vi "TP 2.3 (con variable t).vi"() -> ()   [LabVIEW 2013]
panel:
  in  "Función":T1(ring)
  in  "stop":bool
  out "Waveform Graph":dbl[](graph)
  in  "Amplitud":dbl
  in  "Frecuencia":dbl
  in  "Cantida de Muestras":dbl
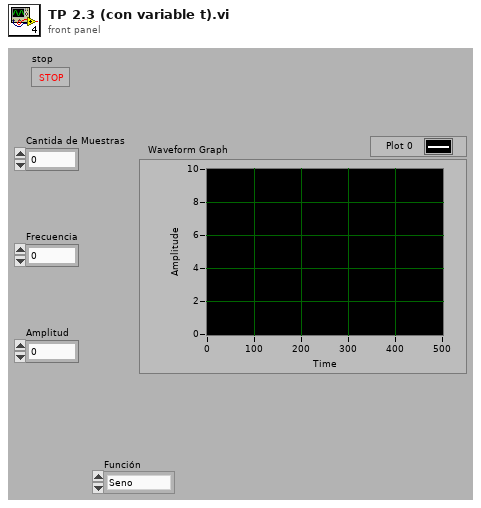
[diagram p1: front panel]
types:
  T1 = enum16{"Seno", "Rampa", "Triangular", "Cuadrada"}
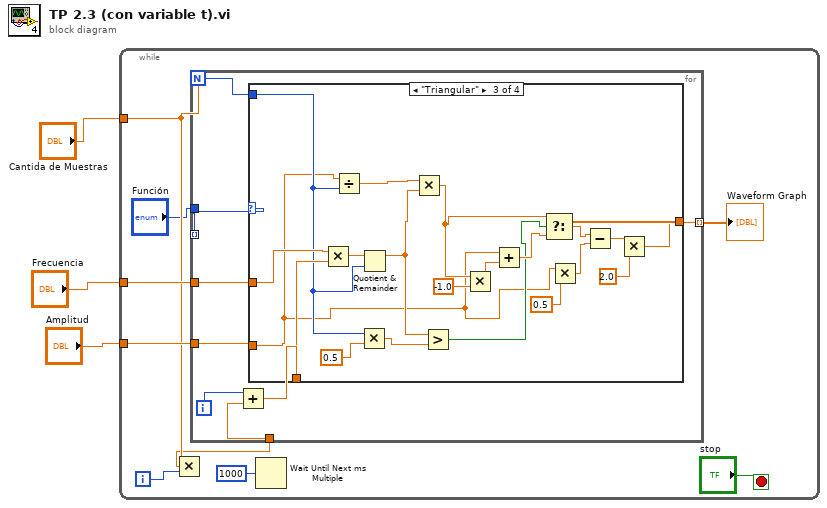
[diagram p0: block diagram]
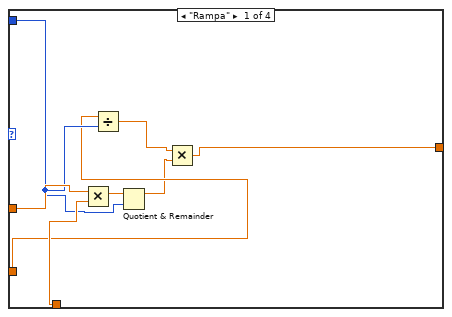
[diagram p2: hidden frame]
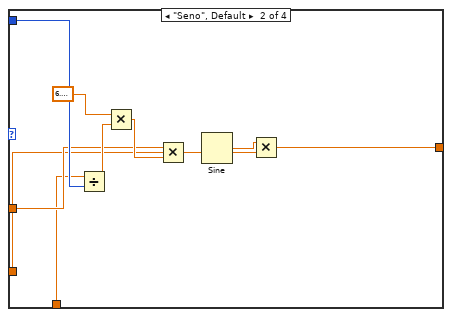
[diagram p3: hidden frame]
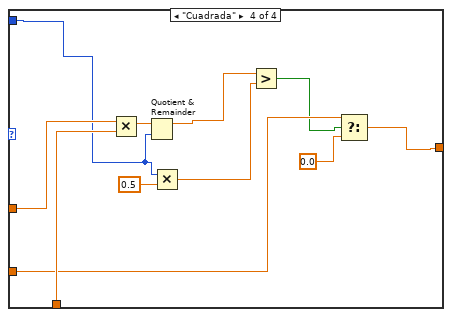
[diagram p4: hidden frame]
diagram:
  n1 = while {
    tunnel: "Cantida de Muestras" -> [w6]
    tunnel: "Frecuencia" -> [w12]
    tunnel: "Amplitud" -> [w11]
    i -> [w7]
    stop <- "stop" stop-if-true
    n2 = Multiply(x=w6, y=w7) -> (x*y=w5:dbl)
    n3 = for {
      N: w6 -> [w20]
      tunnel: w12 -> [w19]
      tunnel: w11 -> [w18]
      tunnel: [w17] -> w10 mode=indexing
      tunnel: w5 -> [w16]
      tunnel: [w13] -> _ mode=indexing
      tunnel: "Función" -> [w13]
      i -> [w15]
      n4 = Add(x=w15, y=w16) -> (x+y=w14:dbl)
      n5 = case shown="\"Triangular\"" w13 {
        tunnel: w20 -> [w25 w38 w47 w59]
        tunnel: w19 -> [w27 w35 w55 w66]
        tunnel: w18 -> [w24 w31 w43 w65]
        tunnel: [w21 w30 w39 w63] -> w17
        tunnel: w14 -> [w28 w29 w56 w67]
        frame "Rampa" {
          n6 = Multiply(x=w27, y=w28) -> (x*y=w26:dbl)
          n7 = Divide(x=w24, y=w25) -> (x/y=w23:dbl)
          n8 = Quotient & Remainder(x=w26, y=w25) -> (x-y*floor(x/y)=w22:dbl)  [unwired: 1 out]
          n9 = Multiply(x=w23, y=w22) -> (x*y=w21:dbl)
        }
        frame "Seno", Default {
          n10 = Divide(x=w29, y=w38) -> (x/y=w37:dbl)
          n11 = Multiply(x=6.283185307179586, y=w37) -> (x*y=w36:dbl)
          n12 = Multiply(x=w35, y=w36) -> (x*y=w33:dbl)
          n13 = Sine(x=w33) -> (sin(x)=w32:dbl)
          n14 = Multiply(x=w32, y=w31) -> (x*y=w30:dbl)
        }
        frame "Triangular" {
          n15 = Multiply(x=w55, y=w56) -> (x*y=w58:dbl)
          n16 = Divide(x=w43, y=w47) -> (x/y=w57:dbl)
          n17 = Multiply(x=w47, y=0.5 ("x")) -> (x*y=w51:dbl)
          n18 = Quotient & Remainder(x=w58, y=w47) -> (x-y*floor(x/y)=w48:dbl)  [unwired: 1 out]
          n19 = Multiply(x=w57, y=w48) -> (x*y=w54:dbl)
          n20 = Greater?(x=w48, y=w51) -> (0:w46:bool)
          n21 = Multiply(x=w54, y=-1.0) -> (x*y=w50:dbl)
          n22 = Add(x=w43, y=w50) -> (x+y=w49:dbl)
          n23 = Select(t=w54, s=w46, f=w49) -> (s? t:f=w45:dbl)
          n24 = Multiply(x=w43, y=0.5 ("x")) -> (x*y=w42:dbl)
          n25 = Subtract(x=w45, y=w42) -> (x-y=w41:dbl)
          n26 = Multiply(x=w41, y=2.0 ("x")) -> (x*y=w39:dbl)
        }
        frame "Cuadrada" {
          n27 = Multiply(x=w66, y=w67) -> (x*y=w68:dbl)
          n28 = Quotient & Remainder(x=w68, y=w59) -> (x-y*floor(x/y)=w60:dbl)  [unwired: 1 out]
          n29 = Multiply(x=w59, y=0.5) -> (x*y=w61:dbl)
          n30 = Greater?(x=w60, y=w61) -> (0:w64:bool)
          n31 = Select(t=w65, s=w64, f=0.0) -> (s? t:f=w63:dbl)
        }
      }
    }
    "Waveform Graph" <- w10
    n32 = Wait Until Next ms Multiple(millisecond multiple=u32 1000) -> ()  [unwired: 1 out]
  }
